vi "Material-ProcessResults-WriteDb.vi"(8 "error in (no error)":errorcluster, 11 "Material-RunTest in":refnum<class "Material-RunTest.lvclass">) -> (0 "error out":errorcluster, 3 "Material-RunTest out":refnum<class "Material-RunTest.lvclass">)   [LabVIEW 2013, in "Material-RunTest.lvclass"]
uses:
  Material-RunTest.lvclass
  Reuse Library/Database API/Database-API.lvclass
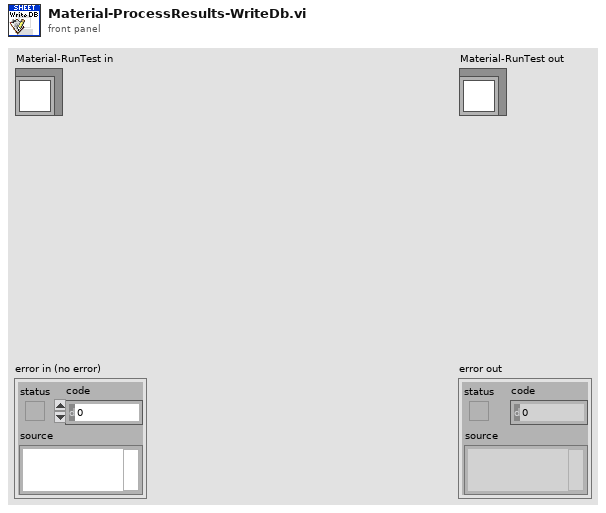
[diagram p1: front panel]
types:
  T1 = cluster{"Lot Number":string, "Line 1 AVG":dbl, "Line 2 AVG":dbl, "Line 3 AVG":dbl, "Value":dbl, string, "Sheet Number":dbl, "seconds since 1Jan1904":timestamp}
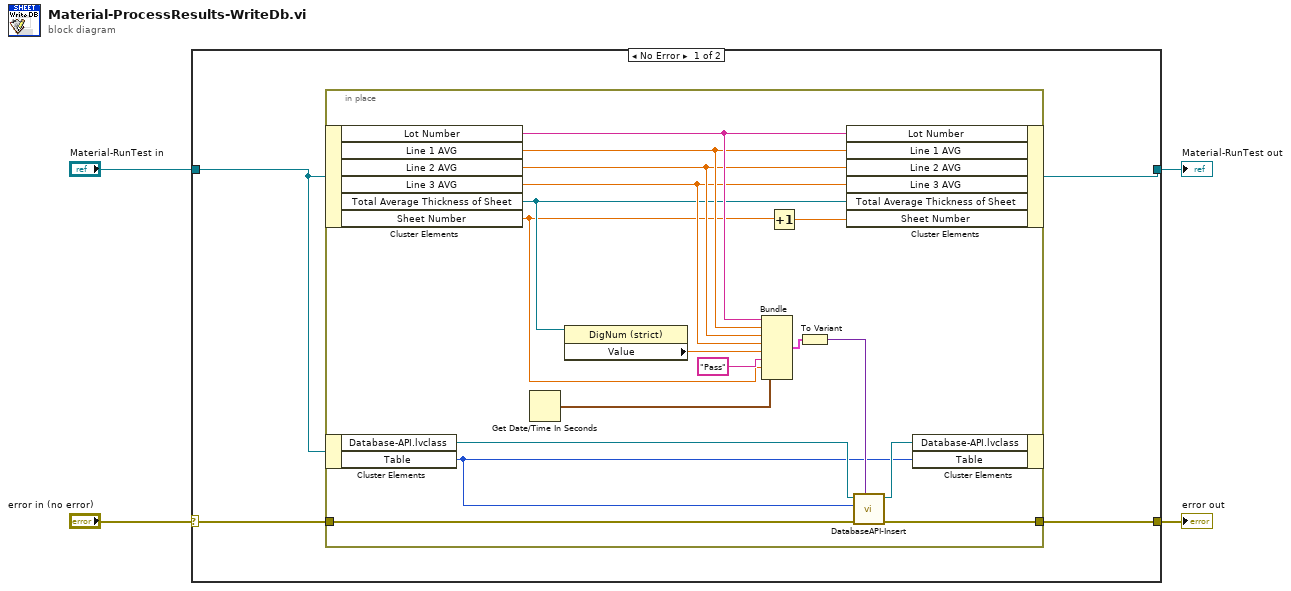
[diagram p0: block diagram]
diagram:
  n1 = case shown="No Error" "error in (no error)" {
    selector: "error in (no error)" -> [w8 w27]
    tunnel: [w6 w27] -> w3
    tunnel: [w5 w26] -> w1
    tunnel: "Material-RunTest in" -> [w7 w26]
    frame No Error {
      n2 = in-place {
        in-place-border: w8 -> [w25]
        in-place-border: [w13] -> w6
        n3 = in-place-cluster #1(w7) -> ("Lot Number"=w21:string, "Line 1 AVG"=w20:dbl, "Line 2 AVG"=w19:dbl, "Line 3 AVG"=w18:dbl, "Total Average Thickness of Sheet"=w17:refnum<vi>, "Sheet Number"=w11:dbl)
        n4 = in-place-cluster #2(w7) -> ("Database-API.lvclass"=w24:refnum<class "Database-API.lvclass">, "Table"=w12:i32)
        n5 = Get Date/Time In Seconds() -> (seconds since 1Jan1904=w9:timestamp)
        n6 = property class="DigNum (strict)"(reference=w17) -> ("Value"=w23:dbl)  [unwired: 1 in, 2 out]
        n7 = Bundle("Lot Number"=w21, "Line 1 AVG"=w20, "Line 2 AVG"=w19, "Line 3 AVG"=w18, "Value"=w23, "Pass", "Sheet Number"=w11, "seconds since 1Jan1904"=w9) -> (w16:T1)  [unwired: 1 in]
        n8 = Increment(x=w11) -> (x+1=w10:dbl)
        n9 = To Variant(anything=w16) -> (Variant=w15:variant)
        n10 = in-place-cluster #1("Lot Number"=w21, "Line 1 AVG"=w20, "Line 2 AVG"=w19, "Line 3 AVG"=w18, "Total Average Thickness of Sheet"=w17, "Sheet Number"=w10) -> (w5:refnum<class "Material-RunTest.lvclass">)
        n11 = call "DatabaseAPI-Insert.vi"("Cluster Data for DB"=w15, "error in (no error)"=w25, "Table"=w12, "Database-API in"=w24) -> ("error out"=w13:errorcluster, "Database-API out"=w14:refnum<class "Database-API.lvclass">)  [unwired: 6 in]
        n12 = in-place-cluster #2("Database-API.lvclass"=w14, "Table"=w12) -> ()  [unwired: 1 out]
      }
    }
    frame Error {
    }
  }
  "error out" <- w3
  "Material-RunTest out" <- w1
